vi "Search Device.vi"(8 "error in":errorcluster, 10 "Device":T2, 11 "Com Port In":T1) -> (0 "error out":errorcluster, 3 "Com Port Out":T1)   [LabVIEW 2018]
uses:
  Data Def/Device.ctl
  Data Def/Com Port.ctl
  <vilib>/Instr/_visa.llb/VISA Find Search Mode.ctl
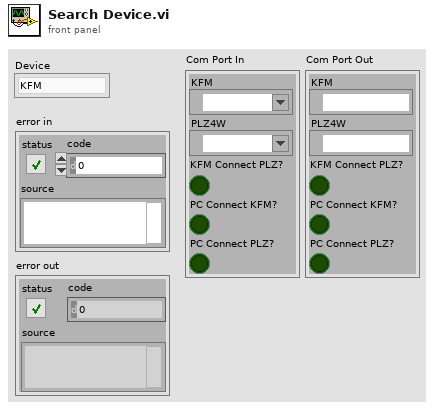
[diagram p1: front panel]
types:
  T1 = typedef "Com Port.ctl" = cluster{"KFM":refnum<visa-resource-name>, "PLZ4W":refnum<visa-resource-name>, "KFM Connect PLZ?":bool, "PC Connect KFM?":bool, "PC Connect PLZ?":bool}
  T2 = typedef "Device.ctl" = enum16{"KFM", "PLZ"}
  T3 = typedef "VISA Find Search Mode.ctl" = u32
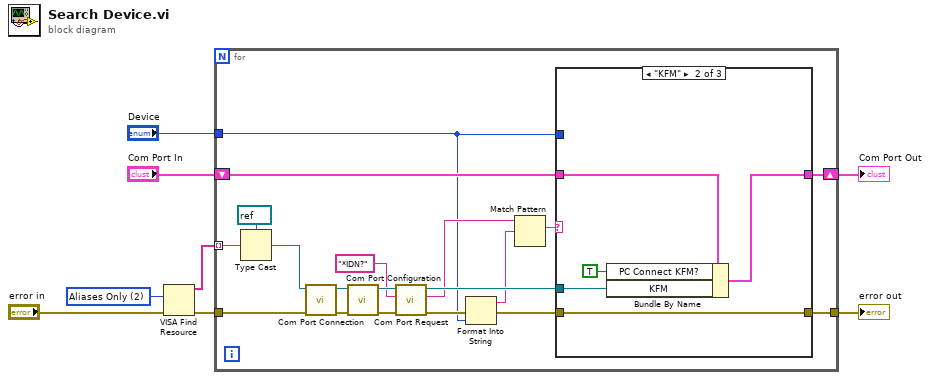
[diagram p0: block diagram]
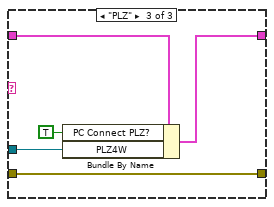
[diagram p3: hidden frame]
diagram:
  w8 = T3 2 items=["Canonical Names Only"=0, "Aliases Only"=2, "Include Matching Aliases"=3, "Include All Aliases"=4] ("Search Mode")
  n1 = VISA Find Resource(8:"error in", 10:w8) -> (0:w6:errorcluster, 3:w5:string[])  [unwired: 1 in, 1 out]
  n2 = for {
    tunnel: w5 -> [w26] mode=indexing
    tunnel: w6 -> [w27]
    shift-right: [w20] -> w2
    shift-left: "Com Port In" -> [w21]
    tunnel: [w19] -> w1
    tunnel: "Device" -> [w9]
    n3 = Type Cast(type=refnum<visa-resource-name> refnum ("Com Port In"), x=w26) -> (*(type *) &x=w24:refnum<visa-resource-name>)
    n4 = call "Com Port Connection.vi"("error in"=w27, "Com Port In"=w24) -> ("error out"=w23:errorcluster, "Com Port Out"=w22:refnum<visa-resource-name>)  [unwired: 8 in]
    n5 = call "Com Port Configuration.vi"("error in"=w23, "Com Port In"=w22) -> ("error out"=w17:errorcluster, "Com Port Out"=w18:refnum<visa-resource-name>)  [unwired: 8 in]
    n6 = call "Com Port Request.vi"("error in"=w17, "Command"="*IDN?" ("ID Query"), "Com Port In"=w18) -> ("error out"=w13:errorcluster, "Respond"=w14:string, "Com Port Out"=w15:refnum<visa-resource-name>)  [unwired: 6 in]
    n7 = Format Into String(error in=w13, w9) -> (resulting string=w12:string, error out=w11:errorcluster)  [unwired: 2 in]
    n8 = Match Pattern(string=w14, regular expression=w12) -> (match substring=w10:string)  [unwired: 1 in, 3 out]
    n9 = case shown="\"KFM\"" w10 {
      tunnel: w11 -> [w28 w31 w36]
      tunnel: w15 -> [_ w33 w38]
      tunnel: w21 -> [w29 w34 w39]
      tunnel: [w29 w32 w37] -> w20
      tunnel: [w28 w31 w36] -> w19
      tunnel: w9 -> [_ _ _]
      frame Default {
      }
      frame "KFM" {
        n10 = Bundle By Name(cluster=w34, "PC Connect KFM?"=TRUE, "KFM"=w33) -> (w32:T1)
      }
      frame "PLZ" {
        n11 = Bundle By Name(cluster=w39, "PC Connect PLZ?"=TRUE, "PLZ4W"=w38) -> (w37:T1)
      }
    }
  }
  "error out" <- w1
  "Com Port Out" <- w2
